vi "Start.vi"(0 "reference in":refnum<class "mmWave instrument.lvclass">, 5 "TX bursts":refnum<class "mmWave data.lvclass">[](array[class]), 7 "sequence":string[](array[string]), 9 "RX acq length":dbl=320000.0 format="%#_6p", 11 "error in (no error)":errorcluster) -> (4 "reference out":refnum<class "mmWave instrument.lvclass">, 15 "error out":errorcluster)   [LabVIEW 2019, in "mmWave instrument.lvclass"]
doc: "Starts insturment operation:"
uses:
  mmWave instrument.lvclass
  mmWave data_class/mmWave data.lvclass
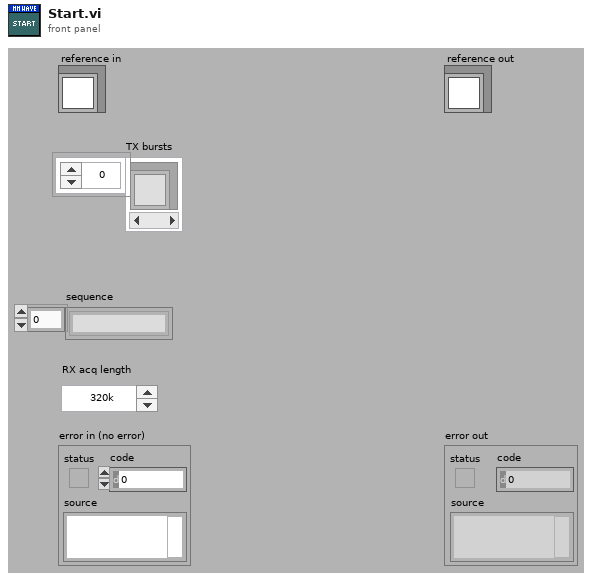
[diagram p1: front panel]
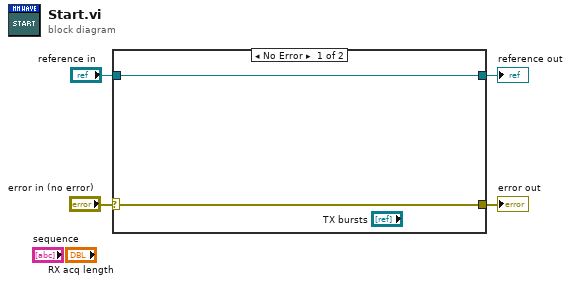
[diagram p0: block diagram]
diagram:
  n1 = case shown="No Error" "error in (no error)" {
    selector: "error in (no error)" -> [w5 w8]
    tunnel: [w5 w8] -> w3
    tunnel: [w6 w7] -> w1
    tunnel: "reference in" -> [w6 w7]
    frame No Error {
    }
    frame Error {
    }
  }
  "error out" <- w3
  "reference out" <- w1
